vi "Hide Unused Subpanels.vi"(8 "error in (no error)":errorcluster, 9 "SubPanels in":refnum<vi>[](array[refnum]), 10 "Used Subpanel Count":i32, 11 "2DArrayManager in":refnum<class "2DArrayManager.lvclass">) -> (0 "error out":errorcluster, 3 "2DArrayManager out":refnum<class "2DArrayManager.lvclass">)   [LabVIEW 2020, in "OOPanel.lvlib" / "2DArrayManager.lvclass"]
uses:
  2DArrayManager.lvclass
  2DArrayManager.lvclass/2DArrayManager.ctl
  Manager/Manager.lvclass
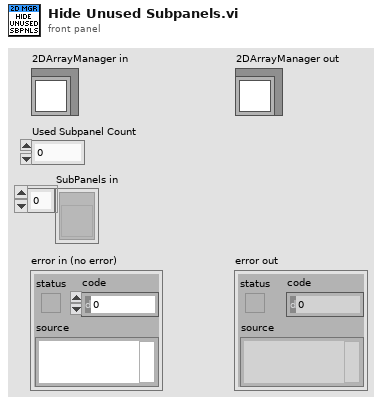
[diagram p1: front panel]
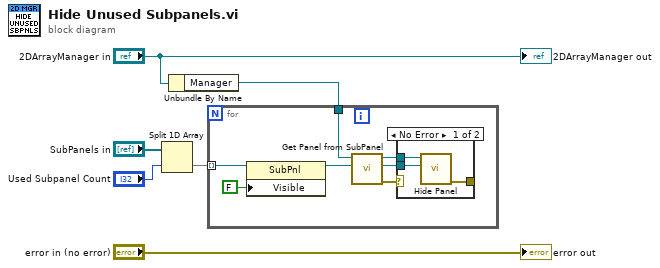
[diagram p0: block diagram]
diagram:
  n1 = Split 1D Array(array="SubPanels in", index="Used Subpanel Count") -> (second subarray=w2:refnum<vi>[])  [unwired: 1 out]
  n2 = Unbundle By Name("2DArrayManager in") -> ("Manager"=w1:refnum<class "Manager.lvclass">)
  n3 = for {
    tunnel: w2 -> [w13] mode=indexing
    tunnel: w1 -> [w10]
    n4 = property class="SubPnl"(reference=w13, "Visible"=FALSE) -> (reference out=w11:refnum<vi>)  [unwired: 1 in, 1 out]
    n5 = call "Get Panel from SubPanel.vi"("SubPanel"=w11, "Manager in"=w10) -> ("error out"=w7:errorcluster, "Panel"=w9:refnum<class "Panel.lvclass">, "Manager out"=w8:refnum<class "Manager.lvclass">)  [unwired: 6 in, 1 out]
    n6 = case shown="No Error" w7 {
      tunnel: w9 -> [w16 _]
      tunnel: w8 -> [w15 _]
      tunnel: [w14 _] -> _
      frame No Error {
        n7 = call "Hide Panel.vi"("Panel In"=w16, "Manager in"=w15) -> ("error out"=w14:errorcluster)  [unwired: 7 in, 2 out]
      }
      frame Error {
      }
    }
  }
  "error out" <- "error in (no error)"
  "2DArrayManager out" <- "2DArrayManager in"
